vi "Automatic Image Scale.vi"(4 "Rotate?":bool, 6 "Box":cluster{"width":sgl, "height":sgl}, 7 "Y offset (point)":sgl, 8 "error in (no error)":errorcluster, 9 "Scale percent IN":sgl, 10 "GetInstanceImage IN":refnum<k24>, 11 "Document":refnum<k24>) -> (0 "error out":errorcluster, 1 "Scale percent OUT":sgl, 2 "GetInstanceImage OUT":refnum<k24>, 3 "Document duplicate":refnum<k24>, 5 "Scaled Image width":sgl)   [LabVIEW 2019, in "Exaprom PDF.lvlib"]
doc: "Version 1.0\nDeveloped by Jean-Marc Simard\nCopyright © 2010, Exaprom Inc.\nAll rights reserved.\nLicense: BSD\n\nWith iTextSharp 4.1.6 (http://itextsharp.sourceforge.net)\nunder Mozilla Public License Version 1.1\n(http://www.mozilla.org/MPL/MPL-1.1.html)"
uses:
  C:/work/niobrara_lv/labview pdf writer fixing/DLL/itextsharp.dll
  DLL/itextsharp.dll
  LV Class/PDF Report Class/PDF Report Class.lvclass
  Exaprom PDF.lvlib
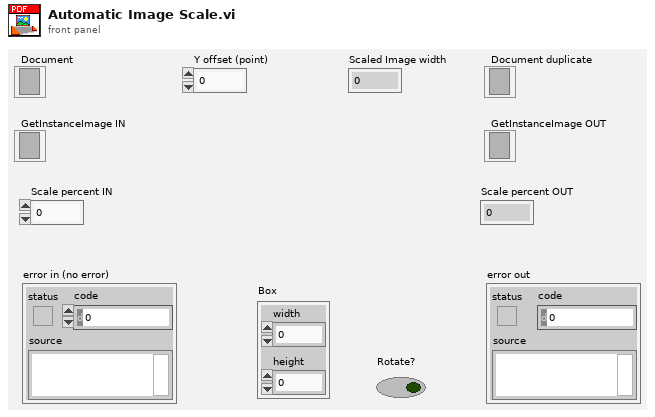
[diagram p1: front panel]
types:
  T1 = typedef "Exaprom PDF.lvlib/Page dimensions.ctl" = cluster{"Start at page":i32, "Page Size":T2, "Orientation":T3, "widht":sgl, "height":sgl, "Margin left":sgl, "Margin right":sgl, "Margin top":sgl, "Margin bottom":sgl, "X0":sgl, "X1":sgl, "Y0":sgl, "Y1":sgl}
  T2 = typedef "Exaprom PDF.lvlib/Page size.ctl" = i32
  T3 = typedef "Exaprom PDF.lvlib/Page Orientation.ctl" = enum16{"Portrait", "Landscape"}
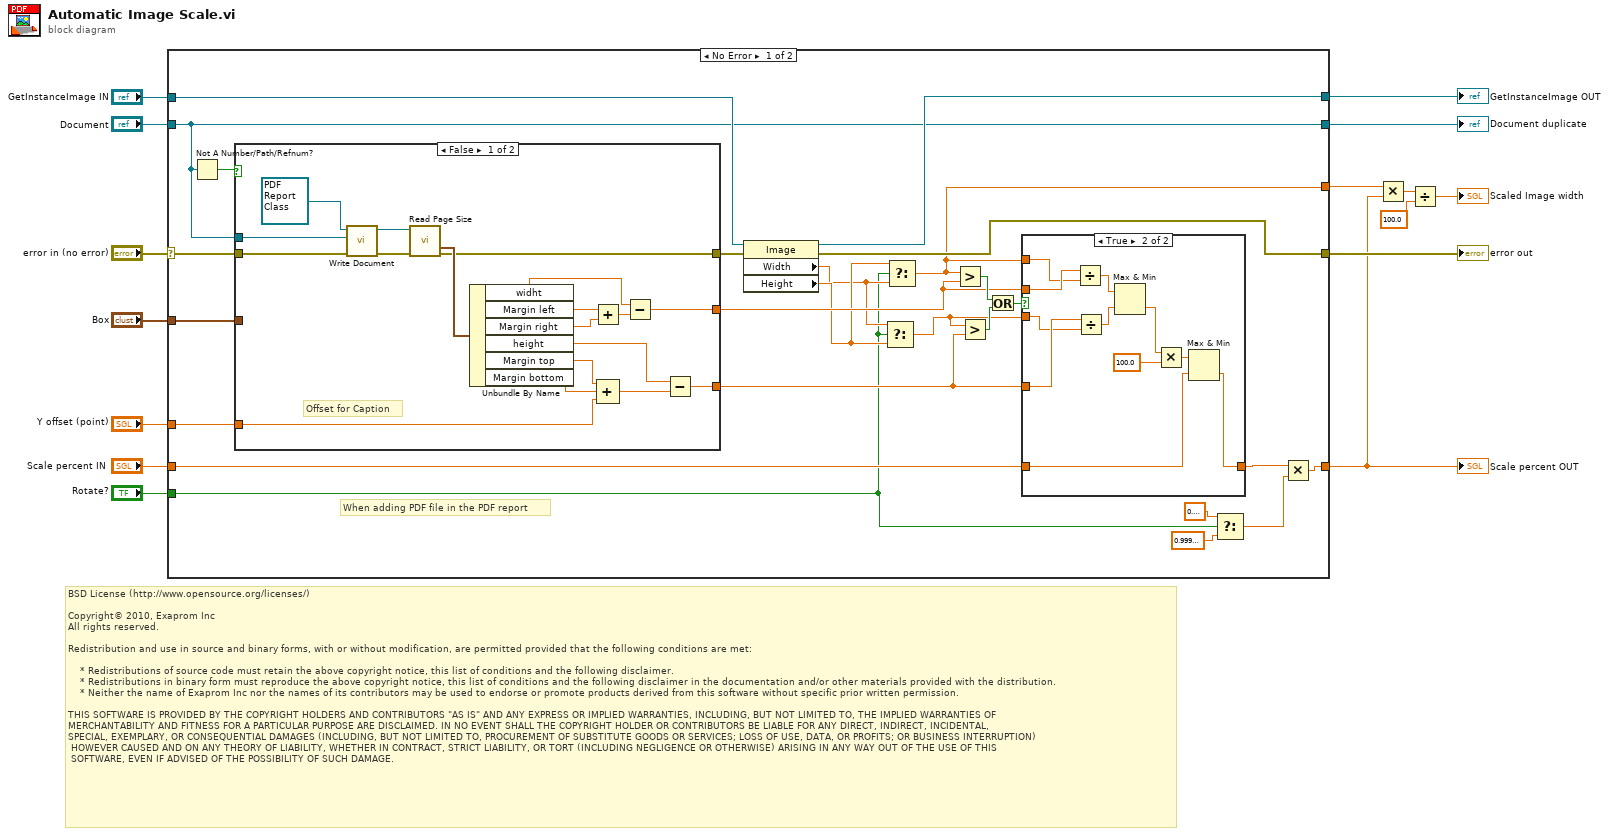
[diagram p0: block diagram]
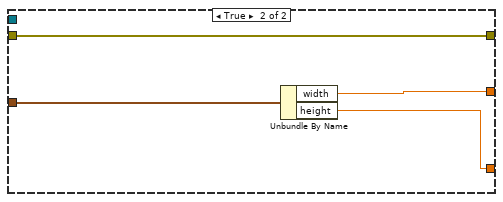
[diagram p2: hidden frame]
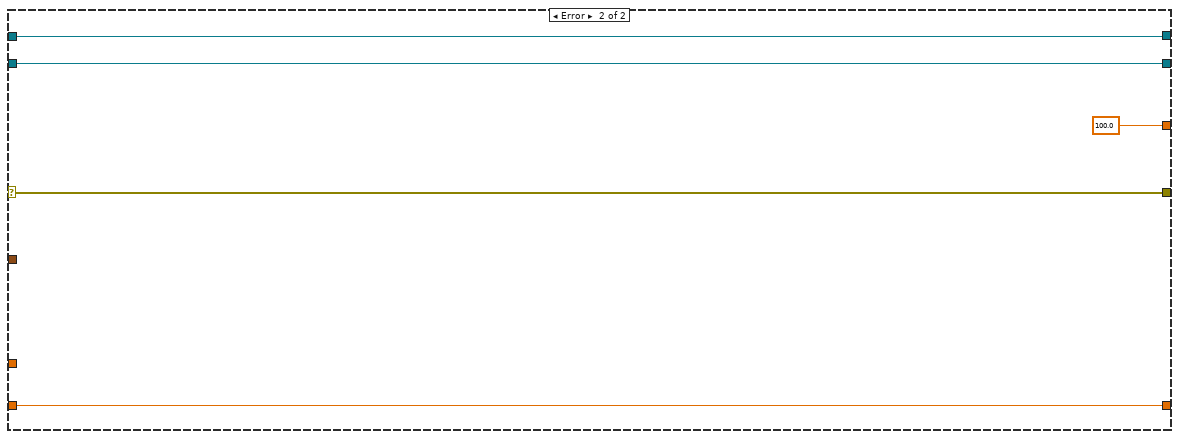
[diagram p4: hidden frame]
diagram:
  # "BSD License (http://www.opensource.org/licenses/)\n\nCopyright© 2010, Exaprom Inc\nAll rights reserved.\n\nRedistribution and use in source and binary forms, with or without modification, are permitted provided that the following conditions are met:\n\n    * Redistributions of source code must retain the above copyright notice, this list of conditions and the following disclaimer.\n    * Redistributions in binary form must reproduce the above copyright notice, this list of conditions and the following disclaimer in the documentation and/or other materials provided with the distribution.\n    * Neither the name of Exaprom Inc nor the names of its contributors may be used to endorse or promote products derived from this software without specific prior written permission.\n\nTHIS SOFTWARE IS PROVIDED BY THE COPYRIGHT HOLDERS AND CONTRIBUTORS \"AS IS\" AND ANY EXPRESS OR IMPLIED WARRANTIES, INCLUDING, BUT NOT LIMITED TO, THE IMPLIED WARRANTIES OF \nMERCHANTABILITY AND FITNESS FOR A PARTICULAR PURPOSE ARE DISCLAIMED. IN NO EVENT SHALL THE COPYRIGHT HOLDER OR CONTRIBUTORS BE LIABLE FOR ANY DIRECT, INDIRECT, INCIDENTAL,\nSPECIAL, EXEMPLARY, OR CONSEQUENTIAL DAMAGES (INCLUDING, BUT NOT LIMITED TO, PROCUREMENT OF SUBSTITUTE GOODS OR SERVICES; LOSS OF USE, DATA, OR PROFITS; OR BUSINESS INTERRUPTION)\n HOWEVER CAUSED AND ON ANY THEORY OF LIABILITY, WHETHER IN CONTRACT, STRICT LIABILITY, OR TORT (INCLUDING NEGLIGENCE OR OTHERWISE) ARISING IN ANY WAY OUT OF THE USE OF THIS\n SOFTWARE, EVEN IF ADVISED OF THE POSSIBILITY OF SUCH DAMAGE."
  n1 = case shown="No Error" "error in (no error)" {
    selector: "error in (no error)" -> [w30 w77]
    tunnel: "GetInstanceImage IN" -> [w40 w79]
    tunnel: "Scale percent IN" -> [w34 w76]
    tunnel: [w25 w76] -> w6
    tunnel: [w28 w78] -> w13
    tunnel: [w33 w79] -> w12
    tunnel: "Document" -> [w28 w78]
    tunnel: [w31 w77] -> w10
    tunnel: "Box" -> [w29 _]
    tunnel: [w23 sgl 100.0 ("Width")] -> w7
    tunnel: "Y offset (point)" -> [w26 _]
    tunnel: "Rotate?" -> [w16 _]
    frame No Error {
      # "When adding PDF file in the PDF report"
      n2 = Not A Number/Path/Refnum?(number/path/refnum=w28) -> (NaN/Path/Refnum?=w32:bool)
      n3 = case shown="False" w32 {
        tunnel: w28 -> [w42 _]
        tunnel: [w46 w62] -> w39
        tunnel: [w56 w60] -> w36
        tunnel: [w55 w59] -> w27
        tunnel: w30 -> [w54 w62]
        tunnel: w29 -> [_ w61]
        tunnel: w26 -> [w45 _]
        frame False {
          # "Offset for Caption"
          n4 = call-dynamic "Write Document.vi"("error in (no error)"=w54, "Document"=w42, "PDF Report Class in"=refnum<class "PDF Report Class.lvclass"> refnum ("PDF Report")) -> ("error out"=w44:errorcluster, "PDF Report Class out"=w41:refnum<class "PDF Report Class.lvclass">)  [unwired: 7 in]
          n5 = call "Read Page Size.vi"("PDF Report"=w41, "error in (no error)"=w44) -> ("Page (points)"=w53:T1, "error out"=w46:errorcluster)  [unwired: 12 out]
          n6 = Unbundle By Name(w53) -> ("widht"=w47:sgl, "Margin left"=w48:sgl, "Margin right"=w49:sgl, "height"=w50:sgl, "Margin top"=w52:sgl, "Margin bottom"=w51:sgl)
          n7 = Add(x=w48, y=w49) -> (x+y=w58:sgl)
          n8 = Compound Arithmetic op=ADD(w52, w51, w45) -> (w57:sgl)
          n9 = Subtract(x=w47, y=w58) -> (x-y=w56:sgl)
          n10 = Subtract(x=w50, y=w57) -> (x-y=w55:sgl)
        }
        frame True {
          n11 = Unbundle By Name(w61) -> ("width"=w60:sgl, "height"=w59:sgl)
        }
      }
      n12 = property class="Image"(reference=w40, error in=w39) -> (reference out=w33:refnum<k24>, error out=w31:errorcluster, "Width"=w20:sgl, "Height"=w21:sgl)
      n13 = Select(t=w20, s=w16, f=w21) -> (s? t:f=w22:sgl)
      n14 = Select(t=w21, s=w16, f=w20) -> (s? t:f=w23:sgl)
      n15 = Greater?(x=w23, y=w36) -> (0:w37:bool)
      n16 = Greater?(x=w22, y=w27) -> (0:w38:bool)
      n17 = Or(x=w37, y=w38) -> (x .or. y?=w35:bool)
      n18 = case shown="True" w35 {
        tunnel: w23 -> [_ w73]
        tunnel: w36 -> [_ w74]
        tunnel: w22 -> [_ w71]
        tunnel: w27 -> [_ w72]
        tunnel: w34 -> [w63 w68]
        tunnel: [w63 w67] -> w24
        frame False {
        }
        frame True {
          n19 = Divide(x=w74, y=w73) -> (x/y=w70:sgl)
          n20 = Divide(x=w72, y=w71) -> (x/y=w69:sgl)
          n21 = Max & Min(x=w70, y=w69) -> (min(x,y)=w65:sgl)  [unwired: 1 out]
          n22 = Multiply(x=w65, y=sgl 100.0) -> (x*y=w66:sgl)
          n23 = Max & Min(x=w66, y=w68) -> (min(x,y)=w67:sgl)  [unwired: 1 out]
        }
      }
      n24 = Select(t=sgl 0.9 ("y"), s=w16, f=sgl 0.999 ("y")) -> (s? t:f=w17:sgl)
      n25 = Multiply(x=w24, y=w17) -> (x*y=w25:sgl)
    }
    frame Error {
    }
  }
  "Scale percent OUT" <- w6
  "Document duplicate" <- w13
  "GetInstanceImage OUT" <- w12
  "error out" <- w10
  n26 = Multiply(x=w7, y=w6) -> (x*y=w5:sgl)
  n27 = Divide(x=w5, y=sgl 100.0) -> (x/y=→"Scaled Image width":sgl)
